vi "test2.vi"() -> ()   [LabVIEW 2017]
uses:
  Detailed Report/Controls/Detailed_Reports_Columns.ctl
  <vilib>/addons/database/Auxilliary.llb/DB Tools Column Info.ctl
  <vilib>/addons/database/Auxilliary.llb/DB Tools DataTypes.ctl
  controls/Mainctrl.ctl
  controls/Main CLuster_Upload.ctl
  SQL/SQL/SQL_DB-Enum.ctl
  <vilib>/addons/database/NI_Database_API.lvlib
panel:
  in  "column information":T1[](array[typedef])=[{"column name"="Barcode", "data type"=enum."String", "size"=100, "allow null?"=TRUE}, {"column name"="Date&Time", "data type"=enum."Date/Time", "size"=50, "allow null?"=TRUE}, {"column name"="User Name", "data type"=enum."String", "size"=100, "allow null?"=TRUE}, {"column name"="Shift", "data type"=enum."String", "size"=10, "allow null?"=TRUE}, {"column name"="Model", "data type"=enum."String", "size"=50, "allow null?"=TRUE}, {"column name"="Variant", "data type"=enum."String", "size"=200, "allow null?"=TRUE}, {"column name"="Test Name", "data type"=enum."String", "size"=1000, "allow null?"=TRUE}, {"column name"="Test Type", "data type"=enum."String", "size"=100, "allow null?"=TRUE}, {"column name"="Excepted Value", "data type"=enum."String", "size"=1000, "allow null?"=TRUE}, {"column name"="HL", "data type"=enum."String", "size"=1000, "allow null?"=TRUE}, {"column name"="LL", "data type"=enum."String", "size"=1000, "allow null?"=TRUE}, {"column name"="Obtained Value", "data type"=enum."String", "size"=1000, "allow null?"=TRUE}, {"column name"="Result", "data type"=enum."String", "size"=20, "allow null?"=TRUE}, {"column name"="Cycle Time", "data type"=enum."String", "size"=50, "allow null?"=TRUE}]
  in  "Column Names":T3=["Barcode", "Date&Time", "User Name", "Shift", "Model", "Variant", "Test Name", "Test Type", "Excepted Value", "HL", "LL", "Obtained Value", "Result", "Cycle Time", "NIP Code"]
  in  "EXIT":bool
  in  "Table Name":string="Detailed_Reports"
  in  "Check and create Table in SQL":bool
  in  "UPLOAD TO CLOUD":bool
  in  "Report Base Path":path
  in  "Connection Info":string="Provider=SQLOLEDB.1;Integrated Security=SSPI;Persist Security Info=False;Initial Catalog=IOT;Data Source=MISPLDESK-SWL04"
  out "error in (no error) 2":errorcluster
  in  "error in (no error)":errorcluster
  # "Report Uploader"
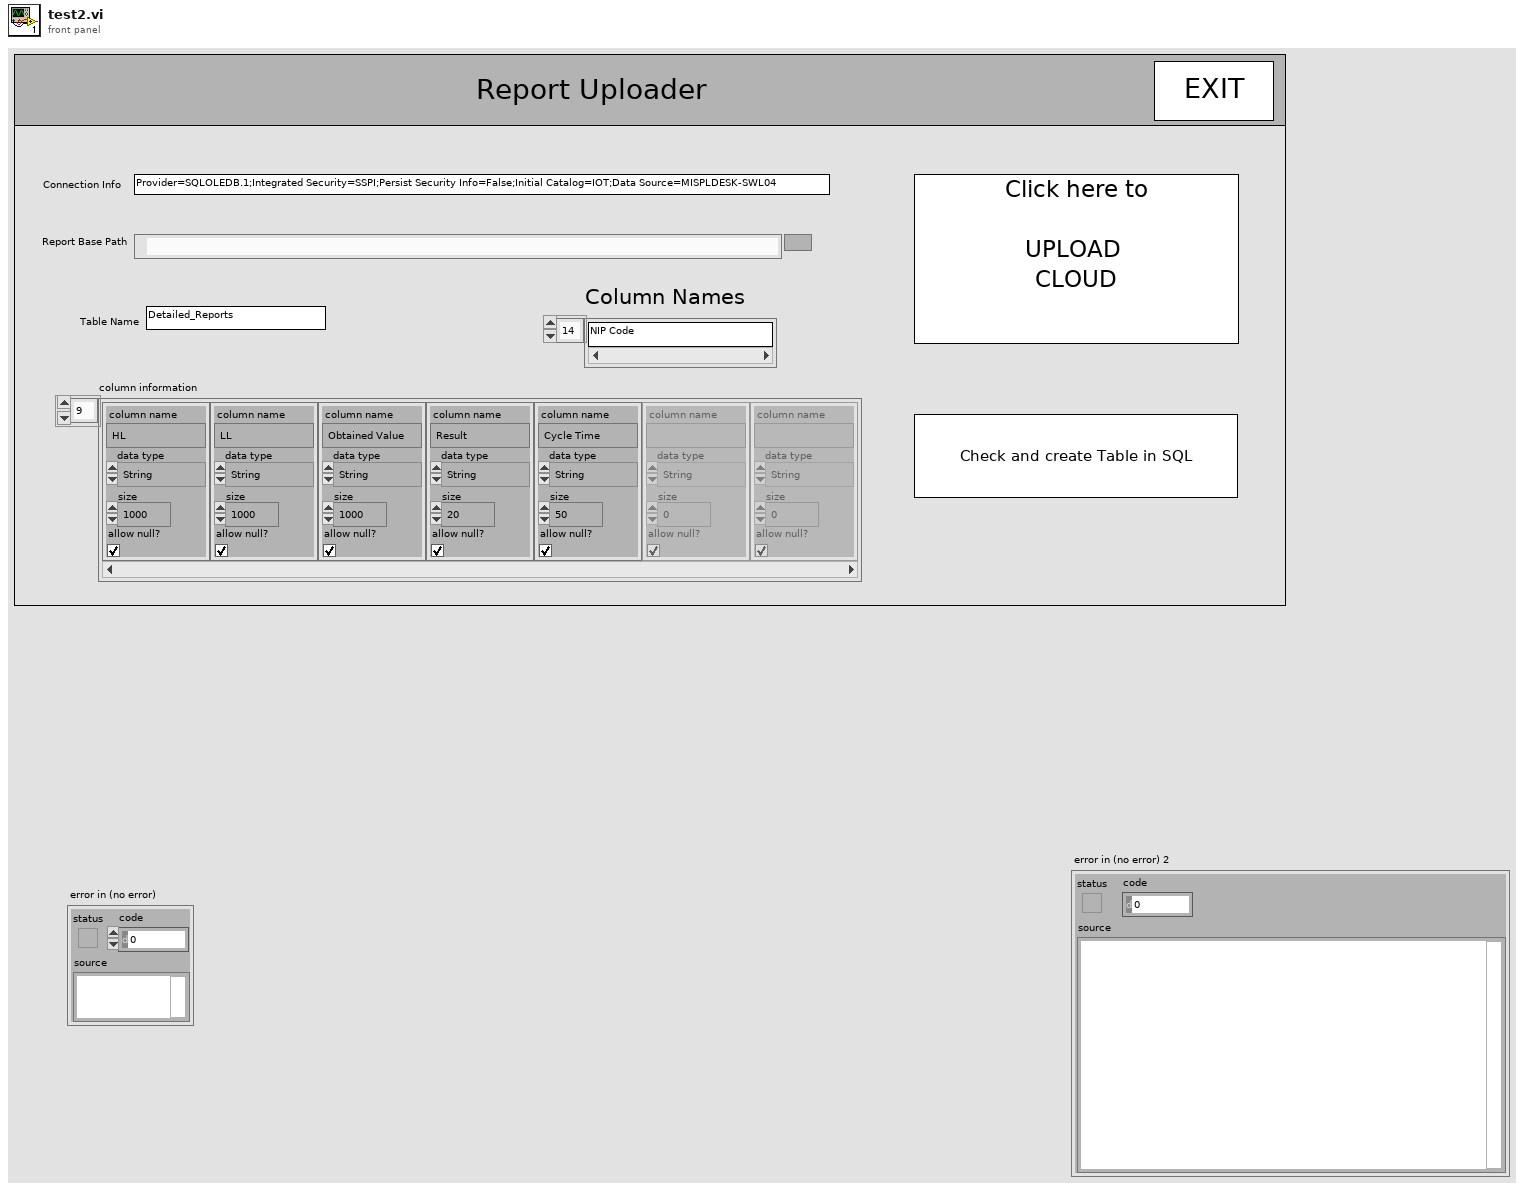
[diagram p1: front panel]
types:
  T1 = typedef "NI_Database_API.lvlib/DB Tools Column Info.ctl" = cluster{"column name":string, "data type":T2, "size":i32, "allow null?":bool}
  T2 = typedef "NI_Database_API.lvlib/DB Tools DataTypes.ctl" = enum16{"String", "Long (I32)", "Single (SGL)", "Double (DBL)", "Date/Time", "Binary"}
  T3 = typedef "Detailed_Reports_Columns.ctl" = string[]
  T4 = typedef "Main CLuster_Upload.ctl" = cluster{"Connectin String":string, "Table Name":string, "Column Names":string[], "column information":T1[]}
  T5 = typedef "Mainctrl.ctl" = enum16{"Check n Create Table", "POLL", "UPLOAD TO SQL", "EXIT", "INI"}
  T6 = cluster{"barcode":string, "Time Stamp":string, "user name":string, "Shift":string, "Model":string, "Variant":string, "Testname":string, "test type":string, "Excepted Value":string, "hl":string, "ll":string, "obtained value":string, "result":string, "cycle time":string, "nip code":string}
  T7 = typedef "SQL_DB-Enum.ctl" = enum16{"INI DATA", "Open Connections", "Query", "Update Table", "Get Full Report", "Get Serial Numbers", "Get Table Columns", "Get Table Names", "Check & Create Table", "Close Connection"}
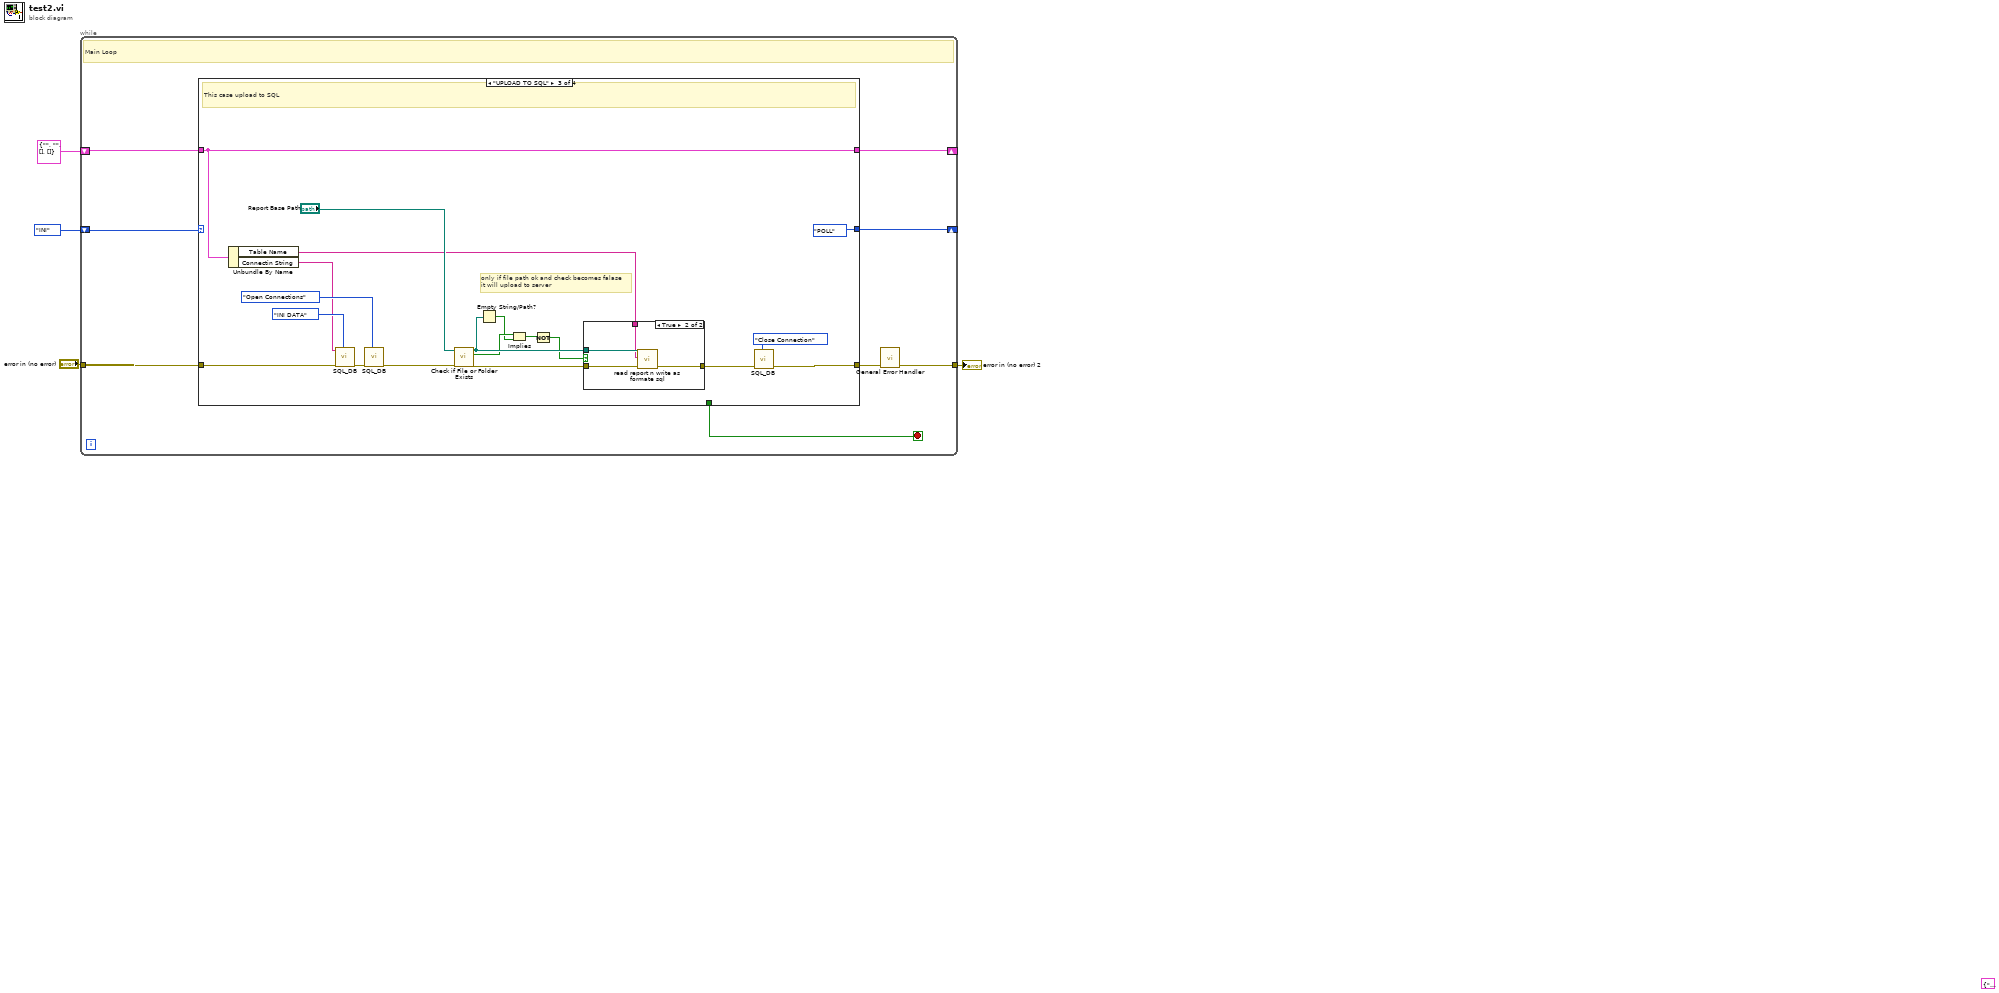
[diagram p0: block diagram]
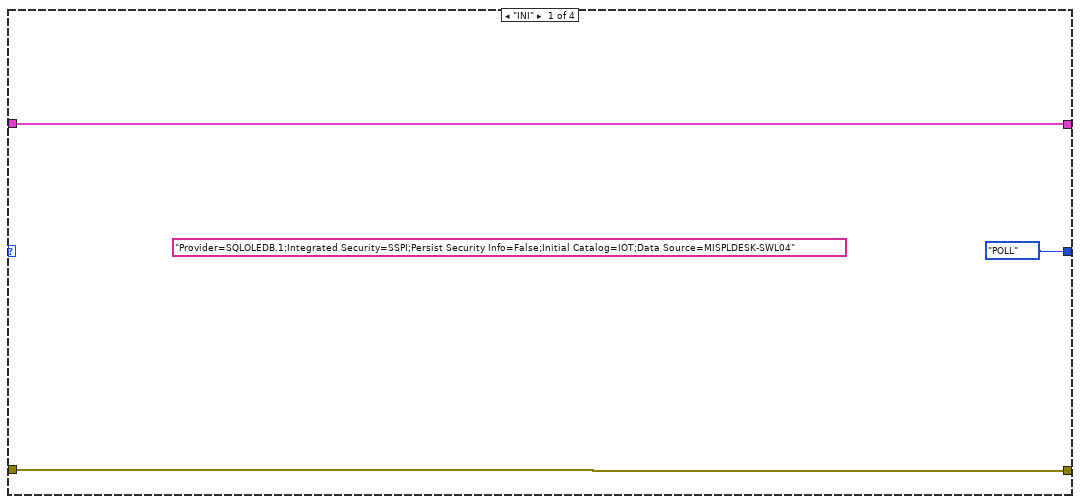
[diagram p2: hidden frame]
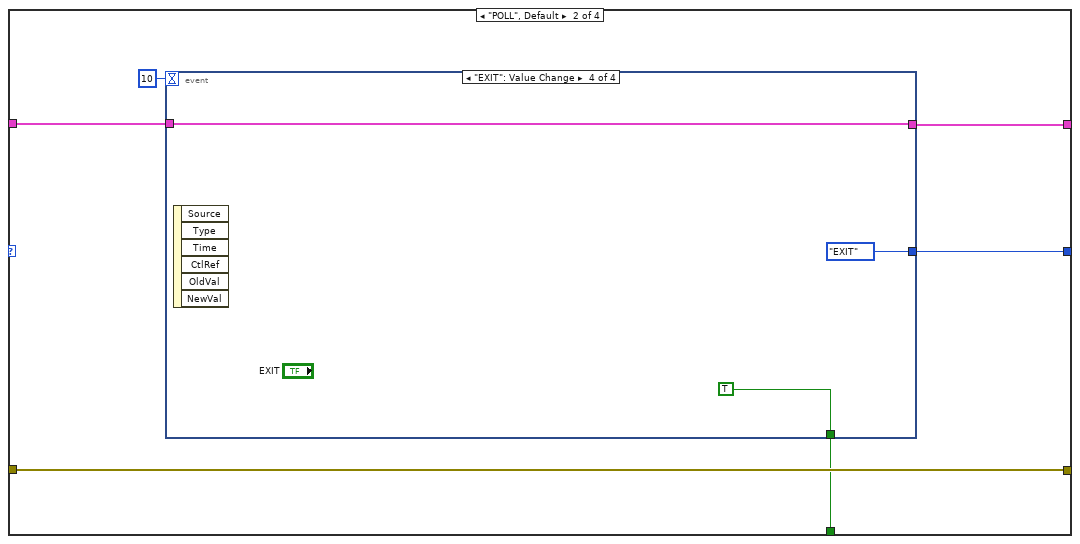
[diagram p3: hidden frame]
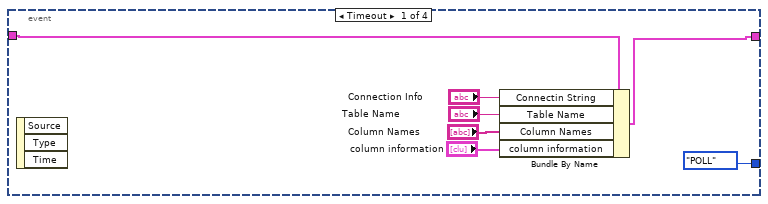
[diagram p4: hidden frame]
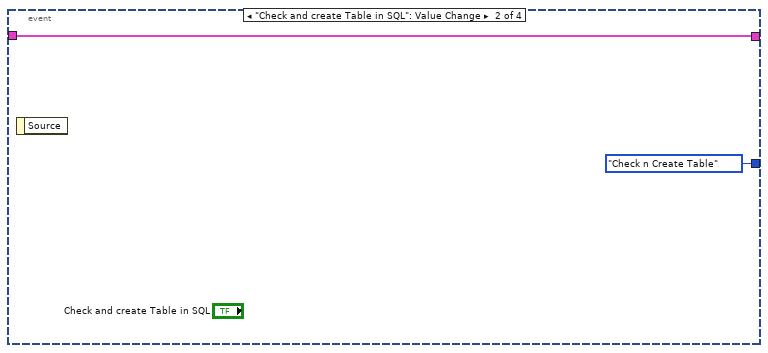
[diagram p5: hidden frame]
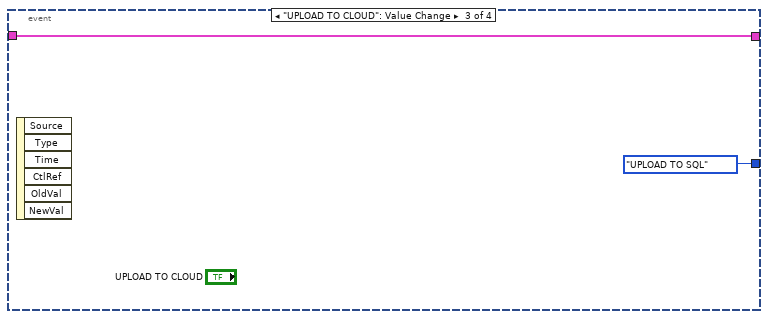
[diagram p6: hidden frame]
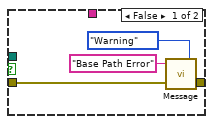
[diagram p7: hidden frame]
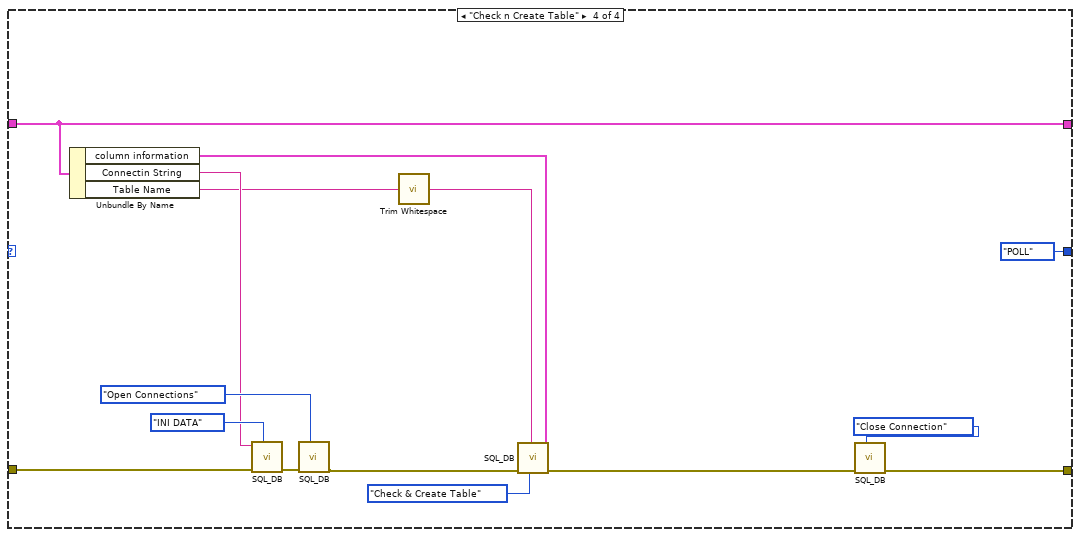
[diagram p8: hidden frame]
diagram:
  (unwired) T6 {"barcode"="barcode", "Time Stamp"="2019-12-13 20:24:09.05", "user name"="1", "Shift"="shifr", "Model"="model", "Variant"="variant", "Testname"="test name", "test type"="test type", "Excepted Value"="test type", "hl"="hl", "ll"="ll", "obtained value"="obtained", "result"="resrut", "cycle time"="Cycle time", "nip code"="nip code"}
  n1 = while {
    shift-right: [w11] -> _
    shift-left: Mainctrl."INI" -> [w12]
    tunnel: "error in (no error)" -> [w10]
    tunnel: [w5] -> w2
    shift-right: [w6] -> _
    shift-left: T4 {"Connectin String"="", "Table Name"="", "Column Names"=[], "column information"=[]} ("Cluster") -> [w7]
    stop <- w8 stop-if-true
    # "Main Loop"
    n2 = case shown="\"UPLOAD TO SQL\"" w12 {
      tunnel: [Mainctrl."POLL" w20 Mainctrl."POLL" Mainctrl."POLL"] -> w11
      tunnel: w10 -> [w13 w19 w37 w73]
      tunnel: [w13 w19 w50 w67] -> w9
      tunnel: [_ w18 _ _] -> w8
      tunnel: w7 -> [w14 w16 w39 w72]
      tunnel: [w14 w17 w39 w72] -> w6
      frame "INI" {
        (unwired) "Provider=SQLOLEDB.1;Integrated Security=SSPI;Persist Security Info=False;Initial Catalog=IOT;Data Source=MISPLDESK-SWL04"
      }
      frame "POLL", Default {
        n3 = event shown="[3] \"EXIT\": Value Change" {
          selector: _ -> [_ _ _ _]
          dyn-events: _ -> [_ _ _ _]
          timeout: 10 -> [_ _ _ _]
          tunnel: [Mainctrl."POLL" Mainctrl."Check n Create Table" Mainctrl."UPLOAD TO SQL" Mainctrl."EXIT"] -> w20
          tunnel: [_ _ _ TRUE] -> w18
          tunnel: [w26 w30 w31 w33] -> w17
          tunnel: w16 -> [w27 w30 w31 w33]
          event Timeout {
            n4 = event-data() -> ()  [unwired: 1 in, 3 out]
            n5 = Bundle By Name(cluster=w27, "Connectin String"="Connection Info", "Table Name"="Table Name", "Column Names"="Column Names", "column information"="column information") -> (w26:T4)
          }
          event "Check and create Table in SQL": Value Change {
            n6 = event-data() -> ()  [unwired: 1 in, 1 out]
          }
          event "UPLOAD TO CLOUD": Value Change {
            n7 = event-data() -> ()  [unwired: 1 in, 6 out]
          }
          event "EXIT": Value Change {
            n8 = event-data() -> ()  [unwired: 1 in, 6 out]
          }
        }
      }
      frame "UPLOAD TO SQL" {
        # "only if file path ok and check becomes falase \nit will upload to server"
        # "This case upload to SQL"
        n9 = Unbundle By Name(w39) -> ("Table Name"=w36:string, "Connectin String"=w38:string)
        n10 = call "SQL_DB.vi"("CTRL"=SQL_DB-Enum."INI DATA", "error in (no error)"=w37, "Connection Info"=w38) -> ("error in (no error) 2"=w41:errorcluster)  [unwired: 6 in, 2 out]
        n11 = call "SQL_DB.vi"("CTRL"=SQL_DB-Enum."Open Connections", "error in (no error)"=w41) -> ("error in (no error) 2"=w40:errorcluster)  [unwired: 7 in, 2 out]
        n12 = call <vilib>:"Check if File or Folder Exists.vi"("error in (no error)"=w40, "path"="Report Base Path") -> ("error out"=w54:errorcluster, "file or folder exists?"=w45:bool, "dup path"=w48:path)  [unwired: 7 in]
        n13 = Empty String/Path?(string/path=w48) -> (empty?=w44:bool)
        n14 = Implies(1:w44, 2:w45) -> (0:w47:bool)
        n15 = Not(x=w47) -> (.not. x?=w46:bool)
        n16 = case shown="True" w46 {
          tunnel: w54 -> [w58 w62]
          tunnel: [w57 w60] -> w52
          tunnel: w48 -> [_ w61]
          tunnel: w36 -> [_ w59]
          frame False {
            n17 = call "Message.vi"("Enum"=enum16{"Error", "Warning", "OK"}."Warning", "error in (no error)"=w58, "Message"="Base Path Error") -> ("error out"=w57:errorcluster)  [unwired: 1 in, 1 out]
          }
          frame True {
            n18 = call "read report n write as formate sql.vi"("error in"=w62, "Table Name"=w59, "file path (dialog if empty)"=w61) -> ("error out"=w60:errorcluster)  [unwired: 8 in]
          }
        }
        n19 = call "SQL_DB.vi"("CTRL"=SQL_DB-Enum."Close Connection", "error in (no error)"=w52) -> ("error in (no error) 2"=w50:errorcluster)  [unwired: 7 in, 2 out]
      }
      frame "Check n Create Table" {
        n20 = Unbundle By Name(w72) -> ("column information"=w63:T1[], "Connectin String"=w71:string, "Table Name"=w64:string)
        n21 = call "SQL_DB.vi"("CTRL"=SQL_DB-Enum."INI DATA", "error in (no error)"=w73, "Connection Info"=w71) -> ("error in (no error) 2"=w69:errorcluster)  [unwired: 6 in, 2 out]
        n22 = call "SQL_DB.vi"("CTRL"=SQL_DB-Enum."Open Connections", "error in (no error)"=w69) -> ("error in (no error) 2"=w70:errorcluster)  [unwired: 7 in, 2 out]
        n23 = call <vilib>:"Trim Whitespace.vi"("string"=w64) -> ("trimmed string"=w76:string)  [unwired: 1 in]
        n24 = call "SQL_DB.vi"("column information"=w63, "Table Name"=w76, "CTRL"=SQL_DB-Enum."Check & Create Table", "error in (no error)"=w70) -> ("error in (no error) 2"=w68:errorcluster)  [unwired: 5 in, 2 out]
        n25 = call "SQL_DB.vi"("CTRL"=SQL_DB-Enum."Close Connection", "error in (no error)"=w68) -> ("error in (no error) 2"=w67:errorcluster)  [unwired: 7 in, 2 out]
      }
    }
    n26 = call <vilib>:"General Error Handler.vi"("error in (no error)"=w9) -> ("error out"=w5:errorcluster)  [unwired: 10 in, 4 out]
  }
  "error in (no error) 2" <- w2
